vi "Read Wrapper for FIFO Type Support.vi"(6 "Timeout (ms)":i32, 7 "Data Element":T4, 8 "error in (no error)":errorcluster, 9 "Read Configuration":T2={"Read Position"=enum."Newest", "Element Offset"=0, "Prepend Array Size"=TRUE, "Get Read Position"=FALSE}, 10 "Data in":u8[](array[numeric]), 11 "CIF_CIPC_Fifo_U8 in":refnum<class "CIF_CIPC_Fifo_U8.lvclass">) -> (0 "error out":errorcluster, 1 "Read Result Details":T1, 2 "Data out":u8[](array[numeric]), 3 "CIF_CIPC_Fifo_U8 out":refnum<class "CIF_CIPC_Fifo_U8.lvclass">, 5 "Success":bool)   [LabVIEW 2021, in "CIF_CIPC_Fifo_U8.lvclass"]
uses:
  CIF_CIPC_Fifo_U8.lvclass
  D:/dev/Packages/CIF_Channels_Core/src/CIFChannels/CIFChannels.lvclass
  D:/dev/Packages/CIF_Channels_Core/src/CIPC_Channels/CIF_CIPC_Chan/CIF_CIPC_Chn.lvclass
  <vilib>/CIF Foundation/CIF CIPC/TypeDefs/Data Element Details.ctl
  <vilib>/CIF Foundation/CIF CIPC/TypeDefs/Read Configuration.ctl
  <vilib>/CIF Foundation/CIF CIPC/TypeDefs/Read Position.ctl
  <vilib>/CIF Foundation/CIF CIPC/TypeDefs/Read Result Details.ctl
  CIFChannels/CIFChannels.lvclass/CIFChannels.ctl
  CIF_CIPC_Chan/CIF_CIPC_Chn.lvclass/CIF_CIPC_Chn.ctl
  CIFChannels/Accessors/Read FIFO Backpressure.vi
  <vilib>/CIF Foundation/CIF CIPC/SubVIs/Wait For N Elements Available.vi
  <vilib>/CIF Foundation/CIF CIPC/SubVIs/Get Element Read Position.vi
  <vilib>/CIF Foundation/CIF CIPC/SubVIs/Check Error.vi
  <vilib>/CIF Foundation/CIF CIPC/SubVIs/Get dll Path.vi
  <vilib>/CIF Foundation/CIF CIPC/SubVIs/Set Element Read Position.vi
  5d919423-ef01-4d49-a0b2-6d9051ec7dc1.vi/331f6ecb-7ec4-4931-b93d-4fbd8d66a851.vi
  5d919423-ef01-4d49-a0b2-6d9051ec7dc1.vi/5ce0d4cf-f921-42ba-b14c-c90f7f7611e4.vi
  <vilib>/CIF Foundation/CIF CIPC/SubVIs/Notify Of New Write.vi
  <vilib>/CIF Foundation/CIF CIPC/SubVIs/Get Element Write Position.vi
  <vilib>/Utility/error.llb/Trim Whitespace.vi
  <vilib>/Utility/error.llb/Error Cluster From Error Code.vi
  <vilib>/CIF Foundation/CIF CIPC/SubVIs/Get Element Info Variant.vi
  CIF_CIPC_Fifo_U8.lvclass/CIF_CIPC_Fifo_U8.ctl
  CIF_CIPC_Chan/CIF_CIPC_Chn.lvclass
  b5615cf0-cd7f-4476-b9a9-d6ef7628cc3b.vi
  6248fc70-cc83-4025-b778-a3221b95feac.vi
  D:/dev/Packages/CIF_Channels_Core/src/CIPC_Channels/FIFO_U8/CIF_CIPC_Fifo_U8.lvclass
  <vilib>/CIF Foundation/CIF CIPC/CIF_NI_CIPC.lvlib
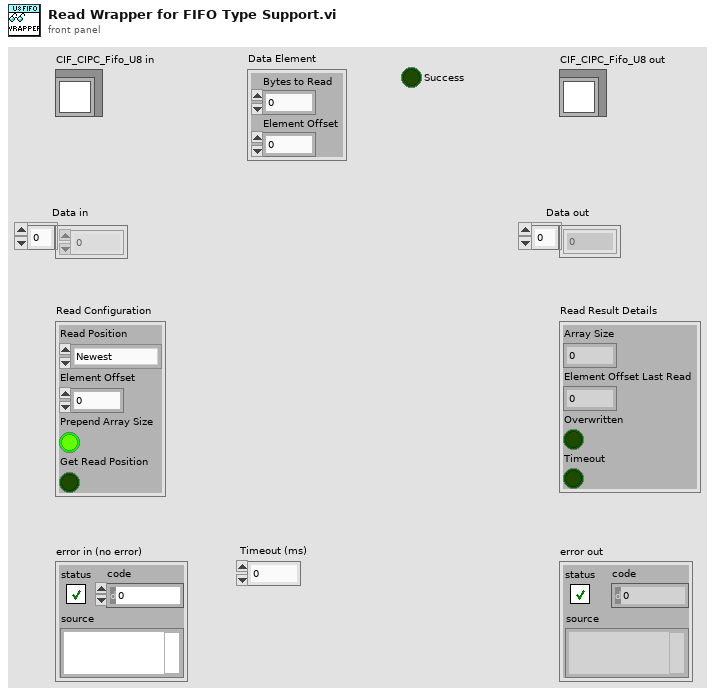
[diagram p1: front panel]
types:
  T1 = typedef "CIF_NI_CIPC.lvlib/Read Result Details.ctl" = cluster{"Array Size":i32, "Element Offset Last Read":u32, "Overwritten":bool, "Timeout":bool}
  T2 = typedef "CIF_NI_CIPC.lvlib/Read Configuration.ctl" = cluster{"Read Position":T3, "Element Offset":i32, "Prepend Array Size":bool, "Get Read Position":bool}
  T3 = typedef "CIF_NI_CIPC.lvlib/Read Position.ctl" = enum16{"Next", "Newest", "Oldest", "Next Available", "Absolute"}
  T4 = typedef "CIF_NI_CIPC.lvlib/Data Element Details.ctl" = cluster{"Bytes to Read":u32, "Element Offset":u32}
  T5 = typedef "CIF_CIPC_Chn.lvclass/Buffer Configuration Data.ctl" = cluster{"Total Size":u32, "Read Size":u32, "Read Offset":u32, "CIPC BP References":T6, "Override CIPC Name":string, "Encoder Data":string}
  T6 = typedef "CIF_NI_CIPC.lvlib/Backpressure References.ctl" = cluster{"CIPC Reference":u64, "CIPC BP Reference":u64}
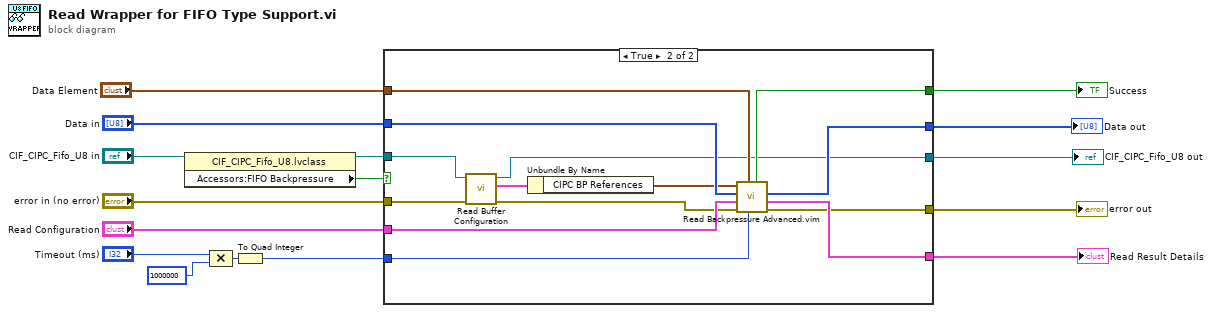
[diagram p0: block diagram]
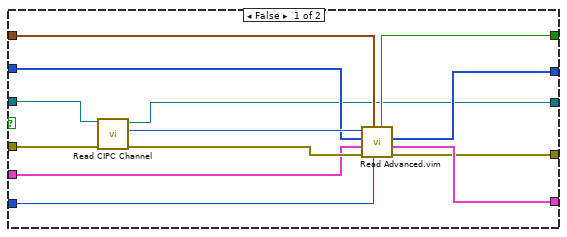
[diagram p2: hidden frame]
diagram:
  n1 = property class="CIF_CIPC_Fifo_U8.lvclass"(reference="CIF_CIPC_Fifo_U8 in") -> (reference out=w15:refnum<class "CIF_CIPC_Fifo_U8.lvclass">, "Accessors:FIFO Backpressure"=w16:bool)  [unwired: 1 in, 1 out]
  n2 = Compound Arithmetic op=MULTIPLY("Timeout (ms)", 1000000 ("value")) -> (w13:i32)
  n3 = To Quad Integer(1:w13) -> (0:w14:i64)
  n4 = case shown="True" w16 {
    tunnel: "Data Element" -> [w27 w43]
    tunnel: "Data in" -> [w26 w42]
    tunnel: "Read Configuration" -> [w25 w41]
    tunnel: [w24 w40] -> w1
    tunnel: [w23 w39] -> w5
    tunnel: [w22 w38] -> w3
    tunnel: [w21 w37] -> w2
    tunnel: "error in (no error)" -> [w20 w34]
    tunnel: w14 -> [w19 w36]
    tunnel: w15 -> [w18 w35]
    tunnel: [w17 w32] -> w4
    frame False {
      n5 = call "Read CIPC Channel.vi"("error in (no error)"=w20, "CIFTag in"=w18) -> ("error out"=w28:errorcluster, "CIPC Channel"=w29:u64, "CIFTag out"=w17:refnum<class "CIF_CIPC_Fifo_U8.lvclass">)  [unwired: 7 in]
      n6 = call "Read Advanced.vim"("Timeout (ns)"=w19, "Data Element"=w27, "error in (no error)"=w28, "Read Configuration"=w25, "Data in"=w26, "CIPC Reference in"=w29) -> ("error out"=w21:errorcluster, "Read Result Details"=w22:T1, "Data out"=w23:u8[], "Success"=w24:bool)  [unwired: 1 in, 1 out]
    }
    frame True {
      n7 = call "Read Buffer Configuration.vi"("error in (no error)"=w34, "CIF_CIPC_Chn in"=w35) -> ("error out"=w33:errorcluster, "Buffer Configuration"=w31:T5, "CIF_CIPC_Chn out"=w32:refnum<class "CIF_CIPC_Fifo_U8.lvclass">)  [unwired: 7 in]
      n8 = Unbundle By Name(w31) -> ("CIPC BP References"=w30:T6)
      n9 = call "Read Backpressure Advanced.vim"("Timeout (ns)"=w36, "Data Element"=w43, "error in (no error)"=w33, "Read Configuration"=w41, "Data in"=w42, "CIPC BP References in"=w30) -> ("error out"=w37:errorcluster, "Read Result Details"=w38:T1, "Data out"=w39:u8[], "Success"=w40:bool)  [unwired: 1 in, 1 out]
    }
  }
  "error out" <- w2
  "CIF_CIPC_Fifo_U8 out" <- w4
  "Success" <- w1
  "Data out" <- w5
  "Read Result Details" <- w3
